vi "UIEnable.vi"(1 "引用":cluster{"数组":refnum<vi>[], "电机":refnum<vi>}) -> ()   [LabVIEW 2018]
uses:
  Device VIs/Verbal.vi
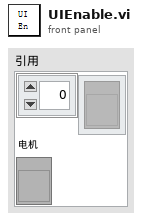
[diagram p1: front panel]
types:
  T1 = enum8{"Enabled", "Disabled", "Disabled and Grayed Out"}
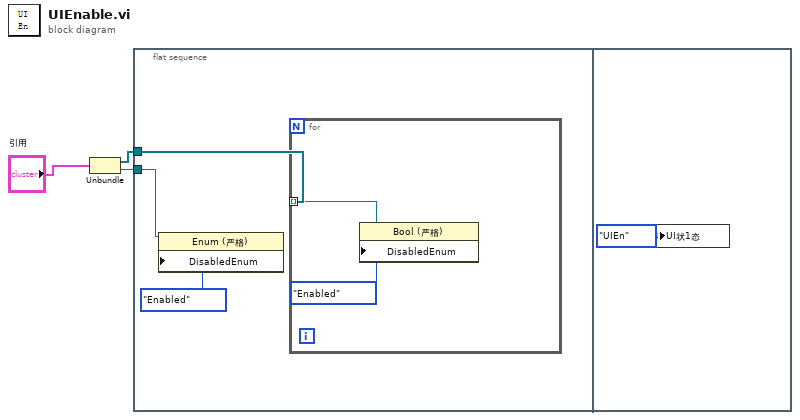
[diagram p0: block diagram]
diagram:
  n1 = Unbundle("引用") -> ("数组"=w3:refnum<vi>[], "电机"=w2:refnum<vi>)
  n2 = flat-sequence {
    tunnel: w3 -> [w6]
    tunnel: w2 -> [w5]
    frame #0 {
      n3 = property class="Enum (严格)"(reference=w5, "DisabledEnum"=T1."Enabled" ("禁用")) -> ()  [unwired: 1 in, 2 out]
      n4 = for {
        tunnel: w6 -> [w8] mode=indexing
        n5 = property class="Bool (严格)"(reference=w8, "DisabledEnum"=T1."Enabled" ("禁用")) -> ()  [unwired: 1 in, 2 out]
      }
    }
    frame #1 {
      n6 = global write "Verbal.vi" "UI状1态"(enum16{"UIEn", "UIDis"}."UIEn" ("UI状态")) -> ()
    }
  }
